vi "test_RS-xxx to GPIB ConvBox Protocol Factory.vi"(8 "error in (no error)":errorcluster, 11 "TestCase in":refnum<class "Instrument Addon Scripting API Protocol Factories Unit Tests.lvclass">) -> (0 "error out":errorcluster, 3 "TestCase out":refnum<class "Instrument Addon Scripting API Protocol Factories Unit Tests.lvclass">)   [LabVIEW 2019, in "Instrument Addon Scripting API Protocol Factories Unit Tests.lvclass"]
uses:
  Instrument Addon Scripting API Protocol Factories Unit Tests.lvclass
  RS-xxx to GPIB ConvBox/RS-xxx to GPIB ConvBox Settings.ctl
  RS-xxx to GPIB ConvBox/RS-xxx to GPIB ConvBox.lvclass
  RS-xxx to GPIB ConvBox/RS-xxx to GPIB ConvBox.lvclass/RS-xxx to GPIB ConvBox.ctl
  RS-xxx to GPIB ConvBox/Data Access/Read Port.vi
  RS-xxx to GPIB ConvBox/Data Access/Read ConvBox Address.vi
  RS-xxx to GPIB ConvBox/Data Access/Read Assert Ren with IFC.vi
  RS-xxx to GPIB ConvBox/Data Access/Read System controller.vi
  RS-xxx to GPIB ConvBox/Data Access/Read IST bit sense.vi
  RS-xxx to GPIB ConvBox/Data Access/Read GPIB Address.vi
  <vilib>/addons/_JKI Toolkits/VI Tester/TestCase.llb/TestCase.lvclass
  C:/Program Files (x86)/National Instruments/LabVIEW 2019/vi.lib/addons/_JKI Toolkits/VI Tester/TestCase.llb/TestCase.lvclass
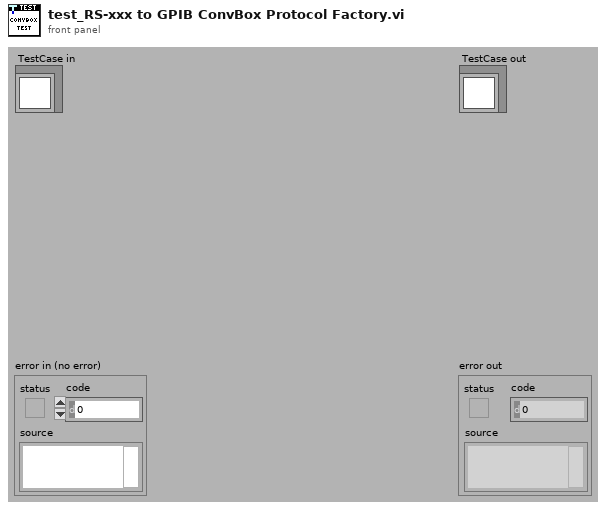
[diagram p1: front panel]
types:
  T1 = typedef "Protocols.lvlib/RS-xxx to GPIB ConvBox.lvclass/RS-xxx to GPIB ConvBox Settings.ctl" = cluster{"Port":string, "ConvBox Address":string, "Assert Ren with IFC":bool, "System Controller":bool, "IST bit sense":bool, "GPIB Address":string}
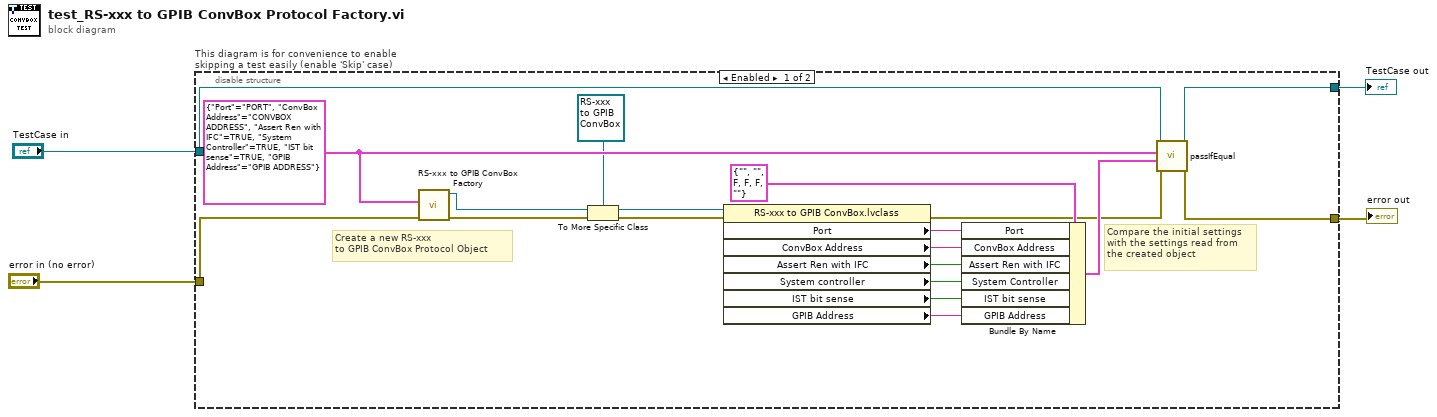
[diagram p0: block diagram]
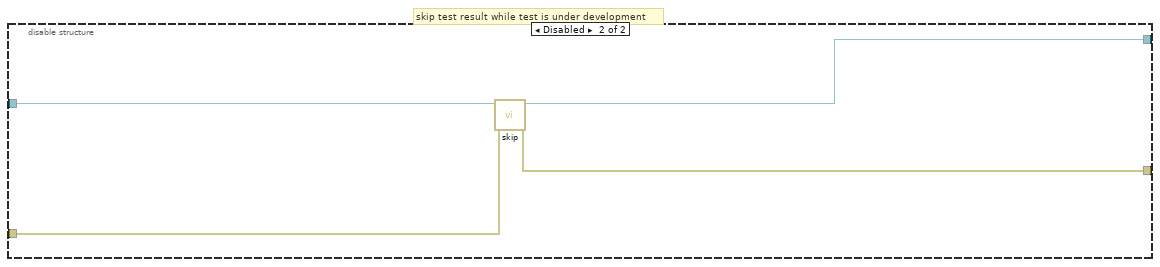
[diagram p2: hidden frame]
diagram:
  n1 = disable-structure "This diagram is for convenience to enable skipping a test easily (enable 'Skip' case)" shown="Enabled" {
    disable-tunnel: "TestCase in" -> [w23 w27]
    disable-tunnel: [w22 w25] -> w1
    disable-tunnel: [w21 w26] -> w3
    disable-tunnel: "error in (no error)" -> [w20 w24]
    frame Enabled {
      w17 = T1 {"Port"="PORT", "ConvBox Address"="CONVBOX ADDRESS", "Assert Ren with IFC"=TRUE, "System Controller"=TRUE, "IST bit sense"=TRUE, "GPIB Address"="GPIB ADDRESS"} ("RS-xxx to GPIB ConvBox settings")
      # "Compare the initial settings \nwith the settings read from \nthe created object"
      # "Create a new RS-xxx \nto GPIB ConvBox Protocol Object"
      n2 = call "RS-xxx to GPIB ConvBox Factory.vi"("error in (no error)"=w20, "RS-xxx to GPIB ConvBox settings"=w17) -> ("error out"=w7:errorcluster, "protocol out"=w6:refnum<class "Protocol Parent.lvclass">)  [unwired: 8 in]
      n3 = To More Specific Class(target class=refnum<class "RS-xxx to GPIB ConvBox.lvclass"> refnum ("Protocols.lvlib:RS-xxx to GPIB ConvBox.lvclass"), reference=w6, error in=w7) -> (specific class reference=w9:refnum<class "RS-xxx to GPIB ConvBox.lvclass">, error out=w8:errorcluster)
      n4 = property class="RS-xxx to GPIB ConvBox.lvclass"(reference=w9, error in=w8) -> (error out=w16:errorcluster, "Port"=w15:string, "ConvBox Address"=w14:string, "Assert Ren with IFC"=w13:bool, "System controller"=w12:bool, "IST bit sense"=w11:bool, "GPIB Address"=w10:string)  [unwired: 1 out]
      n5 = Bundle By Name(cluster=T1 {"Port"="", "ConvBox Address"="", "Assert Ren with IFC"=FALSE, "System Controller"=FALSE, "IST bit sense"=FALSE, "GPIB Address"=""} ("RS-xxx to GPIB ConvBox settings"), "Port"=w15, "ConvBox Address"=w14, "Assert Ren with IFC"=w13, "System Controller"=w12, "IST bit sense"=w11, "GPIB Address"=w10) -> (w18:T1)
      n6 = call-dynamic "passIfEqual.vi"("error in (no error)"=w16, "y"=w18, "x"=w17, "TestCase in"=w23) -> ("error out"=w21:errorcluster, "TestCase out"=w22:refnum<class "Instrument Addon Scripting API Protocol Factories Unit Tests.lvclass">)  [unwired: 6 in]
    }
    frame Disabled {
      # "skip test result while test is under development"
      n7 = call <vilib>:"skip.vi"("error in (no error)"=w24, "TestCase in"=w27) -> ("error out"=w26:errorcluster, "TestCase out"=w25:refnum<class "Instrument Addon Scripting API Protocol Factories Unit Tests.lvclass">)  [unwired: 8 in]
    }
  }
  "error out" <- w3
  "TestCase out" <- w1
